vi "Init_Current.vi"   [LabVIEW 2015]
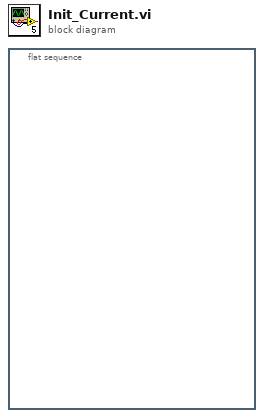
[diagram p0: block diagram]
diagram:
  n1 = flat-sequence {
    frame #0 {
    }
  }
